vi "Teleop.vi"(10 "Match Info":T1={"Autonomous Elapsed Seconds"=0.0, "TeleOp Elapsed Seconds"=0.0, "Disabled Elapsed Seconds"=0.0, "Visited Autonomous"=FALSE, "Visited TeleOp"=FALSE, "Visited Disabled"=FALSE, "Autonomous Settings"={"Autonomous Style"=enum."Independent", "VI Refnum"=refnum}}, 11 "Call Context":T2) -> ()   [LabVIEW 2012]
doc: "This VI is called for each TeleOp packet received from the DS where the robot is not disabled. It is often used to read from the joysticks and update I/O or to update setpoints for timed control loops. It should complete and return within 20 milliseconds or it may miss DS packets."
uses:
  Robot Global Data.vi
  <vilib>/Rock Robotics/WPI/Solenoid/Deprecated/WPI_SolenoidSetBool.vi
  <vilib>/Rock Robotics/WPI/DriverStation/WPI_DriverStationMatch Info.ctl
  <vilib>/Rock Robotics/WPI/DriverStation/WPI_DriverStationDerivedRobotMode.ctl
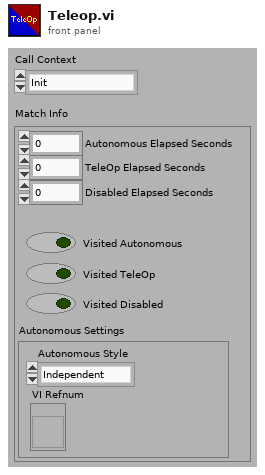
[diagram p1: front panel]
types:
  T1 = typedef "WPI_DriverStationMatch Info.ctl" = cluster{"Autonomous Elapsed Seconds":dbl, "TeleOp Elapsed Seconds":dbl, "Disabled Elapsed Seconds":dbl, "Visited Autonomous":bool, "Visited TeleOp":bool, "Visited Disabled":bool, "Autonomous Settings":cluster{"Autonomous Style":enum16{"Iterative", "Independent"}, "VI Refnum":refnum<vi>}}
  T2 = typedef "WPI_DriverStationDerivedRobotMode.ctl" = enum16{"Init", "Execute", "Stop"}
  T3 = typedef "WPI_DigitalInputDevRef.ctl" = cluster{"DevStatus":errorcluster, "DIO Channel":T4, "Digital Module":T5}
  T4 = typedef "FPGA_DIOChannel.ctl" = enum8{"DIO 1", "DIO 2", "DIO 3", "DIO 4", "DIO 5", "DIO 6", "DIO 7", "DIO 8", "DIO 9", "DIO 10", "DIO 11", "DIO 12", "DIO 13", "DIO 14", "Invalid"}
  T5 = typedef "FPGA_TypedefDigitalModule.ctl" = enum16{"Digital Module 1", "Digital Module 2"}
  T6 = typedef "WPI_MotorControlDeviceRef.ctl" = cluster{"DeviceStatus":errorcluster, "Type":enum16{"PWM", "CAN"}, "PWM":cluster{"Digital Module":T5, "PWM Channel":T7, "DeadBand":T8}, "CAN":cluster{"Device Number":u8, "Control Mode":T9, "Semaphore":T10, "Max Vout":dbl}, "Invert":bool, "TransformRef":T11, "InvTransformRef":T11}
  T7 = typedef "FPGA_DIOPWMChannel.ctl" = enum8{"PWM 1", "PWM 2", "PWM 3", "PWM 4", "PWM 5", "PWM 6", "PWM 7", "PWM 8", "PWM 9", "PWM 10", "Invalid"}
  T8 = typedef "WPI_PWMDeadband.ctl" = cluster{"Name":string, "maxPositivePwm":i32, "minPositivePwm":i32, "centerPwm":i32, "maxNegativePwm":i32, "minNegativePwm":i32, "angularRange":u16}
  T9 = typedef "WPI_CANJaguar_ControlMode.ctl" = enum8{"Percent VBus", "Current", "Speed", "Position", "Voltage"}
  T10 = typedef "Semaphore RefNum" = refnum<k1>
  T11 = typedef "WPI_PWMTransform_ConPane.ctl" = refnum<vi>
  T12 = typedef "WPI_JoystickDevRef.ctl" = cluster{"Device":T13}
  T13 = typedef "WPI_JoystickDeviceEnum.ctl" = enum16{"USB 1", "USB 2", "USB 3", "USB 4", "Kinect 1", "Kinect 2"}
  T14 = typedef "WPI_JoystickButtonState.ctl" = cluster{"Button 1":bool, "Button 2":bool, "Button 3":bool, "Button 4":bool, "Button 5":bool, "Button 6":bool, "Button 7":bool, "Button 8":bool, "Button 9":bool, "Button 10":bool, "Button 11":bool, "Button 12":bool}
  T15 = cluster{"axis 1 (x)":dbl, "axis 2 (y)":dbl, "axis 3 (throttle)":dbl, "axis 4":dbl, "axis 5":dbl, "axis 6":dbl}
  T16 = typedef "WPI_RobotDriveDevRef.ctl" = cluster{"DevStatus":errorcluster, "Motors[]":T6[], "Square Inputs":bool, "Max Output":dbl, "Isochronous":bool}
  T17 = typedef "WPI_SolenoidDevRef.ctl" = cluster{"DevStatus":errorcluster, "Solenoid Module":T18, "Forward Solenoid Channel":T19, "Reverse Solenoid Channel":T19}
  T18 = typedef "FPGA_TypedefSolenoidModule.ctl" = enum16{"Solenoid Module 1", "Solenoid Module 2"}
  T19 = typedef "WPI_SolenoidChannel.ctl" = enum8{"Solenoid 1", "Solenoid 2", "Solenoid 3", "Solenoid 4", "Solenoid 5", "Solenoid 6", "Solenoid 7", "Solenoid 8", "Invalid"}
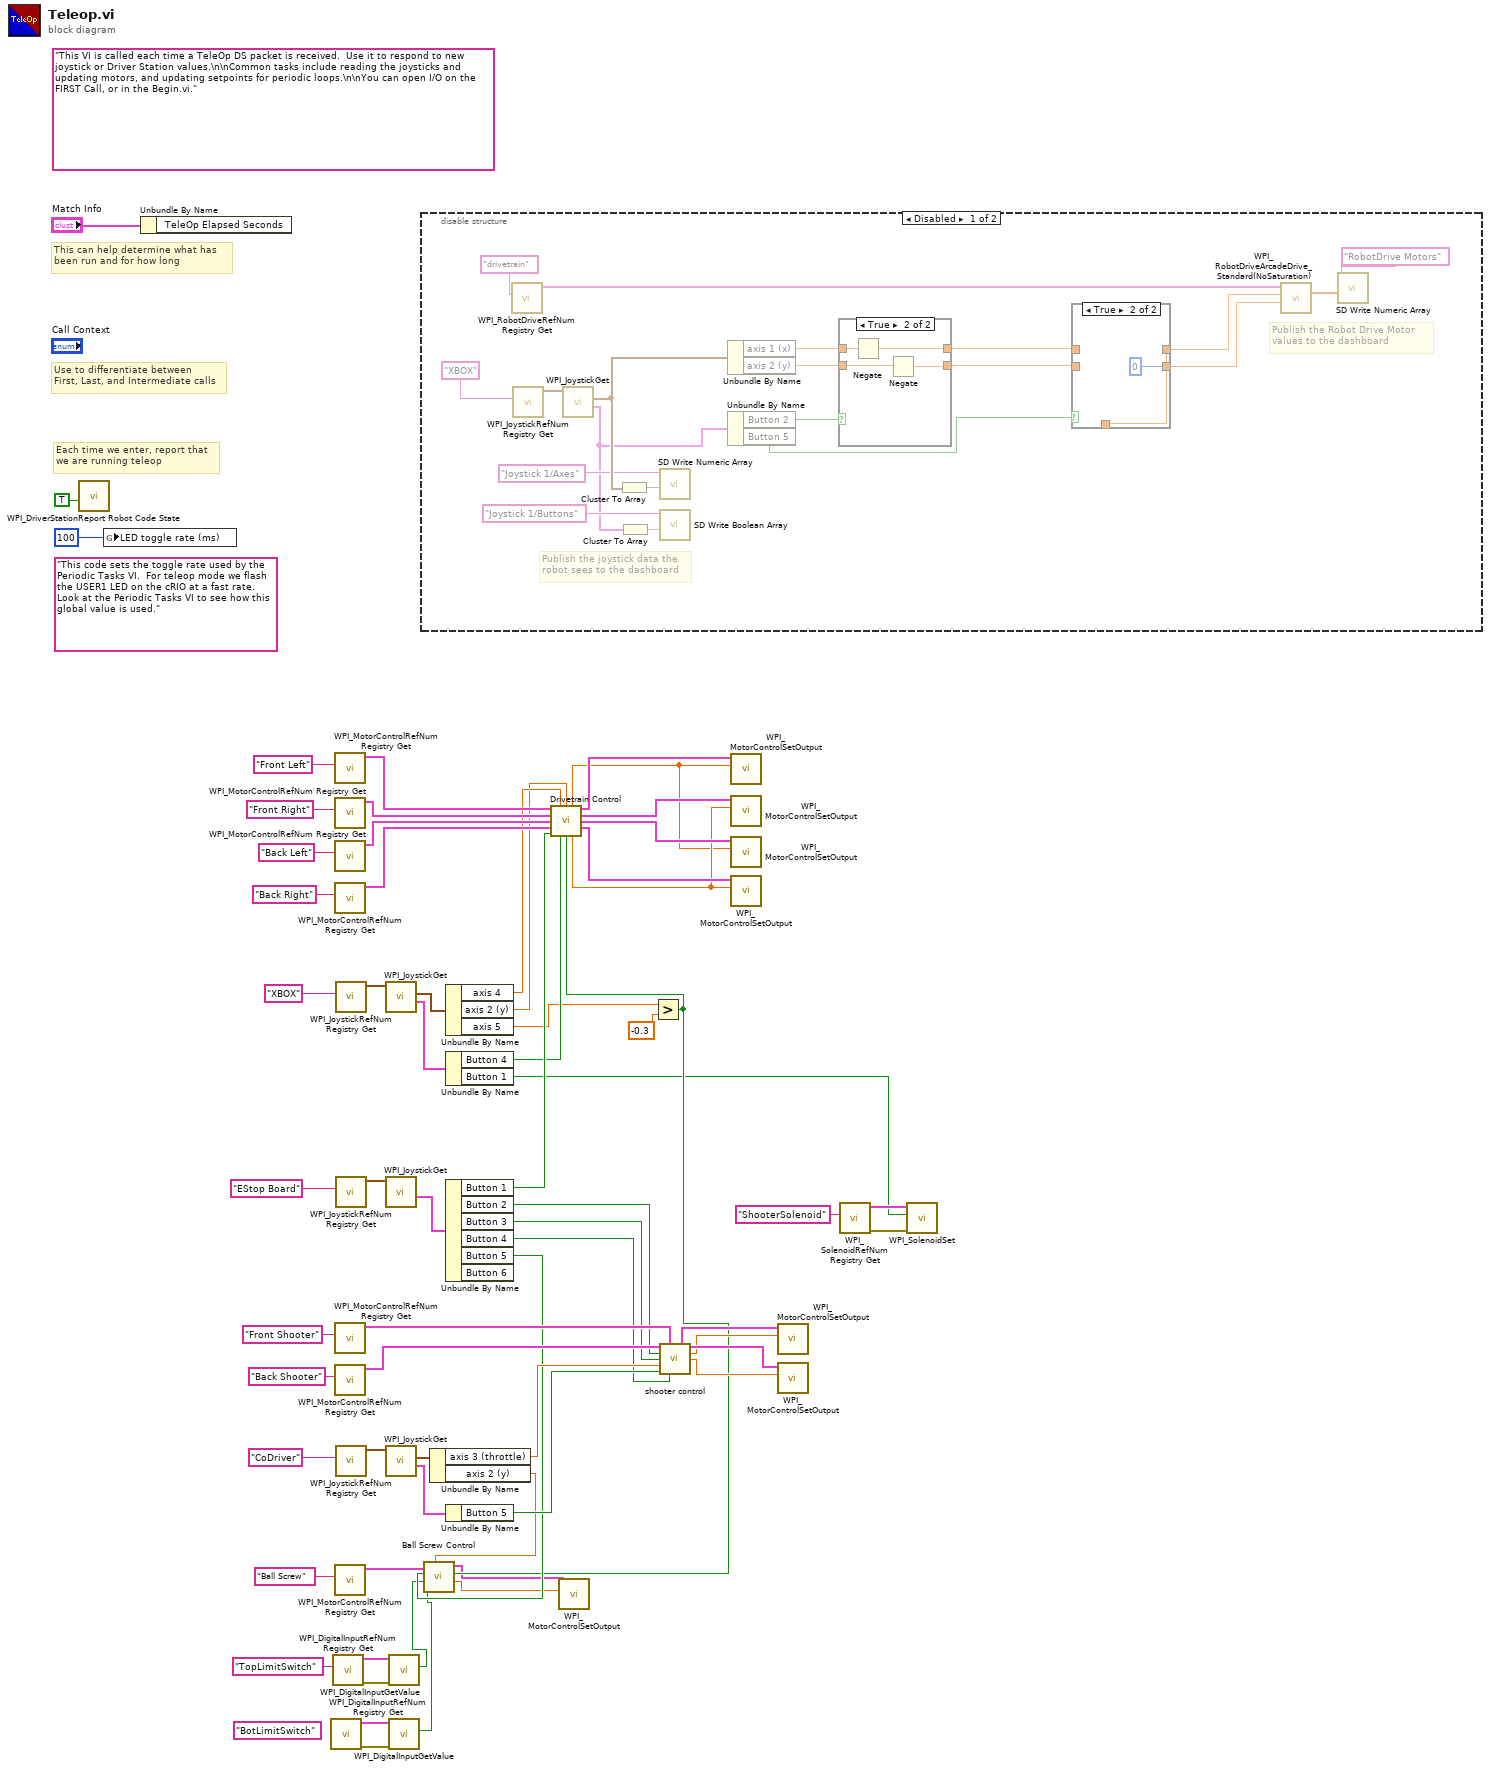
[diagram p0: block diagram]
diagram:
  (unwired) "BotLimitSwitch" ("refnum name")
  (unwired) "This code sets the toggle rate used by the Periodic Tasks VI.  For teleop mode we flash the USER1 LED on the cRIO at a fast rate.  Look at the Periodic Tasks VI to see how this global value is used."
  (unwired) "This VI is called each time a TeleOp DS packet is received.  Use it to respond to new joystick or Driver Station values.\n\nCommon tasks include reading the joysticks and updating motors, and updating setpoints for periodic loops.\n\nYou can open I/O on the FIRST Call, or in the Begin.vi."
  # "Each time we enter, report that\nwe are running teleop"
  # "Use to differentiate between\nFirst, Last, and Intermediate calls"
  # "This can help determine what has\nbeen run and for how long"
  n1 = call <vilib>:"WPI_DriverStationReport Robot Code State.vi"("TeleOp"=TRUE ("Autonomous")) -> ()  [unwired: 10 in, 1 out]
  n2 = global write "Robot Global Data.vi" "LED toggle rate (ms)"(u32 100 ("LED ms toggle rate")) -> ()
  n3 = Unbundle By Name("Match Info") -> ()  [unwired: 1 out]
  n4 = call <vilib>:"WPI_DigitalInputRefNum Registry Get.vi"() -> ("error out"=w14:errorcluster, "DigitalInputDevRef"=w13:T3)  [unwired: 10 in]
  n5 = call <vilib>:"WPI_DigitalInputRefNum Registry Get.vi"("refnum name"="TopLimitSwitch") -> ("error out"=w16:errorcluster, "DigitalInputDevRef"=w15:T3)  [unwired: 9 in]
  n6 = call <vilib>:"WPI_MotorControlRefNum Registry Get.vi"("refnum name"="Front Left") -> ("MotorControlDevRef"=w55:T6)  [unwired: 9 in, 1 out]
  n7 = call <vilib>:"WPI_MotorControlRefNum Registry Get.vi"("refnum name"="Front Right") -> ("MotorControlDevRef"=w54:T6)  [unwired: 9 in, 1 out]
  n8 = call <vilib>:"WPI_MotorControlRefNum Registry Get.vi"("refnum name"="Back Left") -> ("MotorControlDevRef"=w53:T6)  [unwired: 9 in, 1 out]
  n9 = call <vilib>:"WPI_MotorControlRefNum Registry Get.vi"("refnum name"="Back Right") -> ("MotorControlDevRef"=w52:T6)  [unwired: 9 in, 1 out]
  n10 = call <vilib>:"WPI_MotorControlRefNum Registry Get.vi"("refnum name"="Front Shooter") -> ("MotorControlDevRef"=w30:T6)  [unwired: 9 in, 1 out]
  n11 = call <vilib>:"WPI_MotorControlRefNum Registry Get.vi"("refnum name"="Back Shooter") -> ("MotorControlDevRef"=w31:T6)  [unwired: 9 in, 1 out]
  n12 = call <vilib>:"WPI_MotorControlRefNum Registry Get.vi"("refnum name"="Ball Screw") -> ("MotorControlDevRef"=w18:T6)  [unwired: 9 in, 1 out]
  n13 = call <vilib>:"WPI_JoystickRefNum Registry Get.vi"("refnum name"="XBOX") -> ("JoystickDevRef"=w50:T12)  [unwired: 1 in, 9 out]
  n14 = call <vilib>:"WPI_JoystickRefNum Registry Get.vi"("refnum name"="EStop Board") -> ("JoystickDevRef"=w40:T12)  [unwired: 1 in, 9 out]
  n15 = call <vilib>:"WPI_JoystickRefNum Registry Get.vi"("refnum name"="CoDriver") -> ("JoystickDevRef"=w44:T12)  [unwired: 1 in, 9 out]
  n16 = call <vilib>:"WPI_JoystickGet.vi"("JoystickDevRef"=w50) -> ("Buttons"=w46:T14, "Axes"=w49:T15)  [unwired: 1 in, 4 out]
  n17 = call <vilib>:"WPI_JoystickGet.vi"("JoystickDevRef"=w40) -> ("Buttons"=w39:T14)  [unwired: 1 in, 5 out]
  n18 = call <vilib>:"WPI_JoystickGet.vi"("JoystickDevRef"=w44) -> ("Buttons"=w42:T14, "Axes"=w43:T15)  [unwired: 1 in, 4 out]
  n19 = call <vilib>:"WPI_DigitalInputGetValue.vi"("error in (no error)"=w16, "DigitalInputDevRef"=w15) -> ("Value"=w12:bool)  [unwired: 7 in, 2 out]
  n20 = call <vilib>:"WPI_DigitalInputGetValue.vi"("error in (no error)"=w14, "DigitalInputDevRef"=w13) -> ("Value"=w11:bool)  [unwired: 7 in, 2 out]
  n21 = disable-structure shown="Disabled" {
    frame Disabled {
      # "Publish the Robot Drive Motor\nvalues to the dashboard"
      # "Publish the joystick data the\nrobot sees to the dashboard"
      n22 = call <vilib>:"WPI_RobotDriveRefNum Registry Get.vi"("refnum name"="drivetrain") -> ("RobotDriveDevRef"=w85:T16)  [unwired: 1 in, 9 out]
      n23 = call <vilib>:"WPI_JoystickRefNum Registry Get.vi"("refnum name"="XBOX") -> ("JoystickDevRef"=w83:T12)  [unwired: 1 in, 9 out]
      n24 = call <vilib>:"WPI_JoystickGet.vi"("JoystickDevRef"=w83) -> ("Buttons"=w75:T14, "Axes"=w80:T15)  [unwired: 1 in, 4 out]
      n25 = Cluster To Array(cluster=w80) -> (array=w79:dbl[])
      n26 = Cluster To Array(cluster=w75) -> (array=w82:bool[])
      n27 = call <vilib>:"SD Write Numeric Array.vi"("Numeric Array"=w79, "Name"="Joystick 1/Axes") -> ()  [unwired: 8 in, 2 out]
      n28 = call <vilib>:"SD Write Boolean Array.vi"("Boolean Array"=w82, "Name"="Joystick 1/Buttons") -> ()  [unwired: 8 in, 2 out]
      n29 = Unbundle By Name(w80) -> ("axis 1 (x)"=w73:dbl, "axis 2 (y)"=w72:dbl)
      n30 = Unbundle By Name(w75) -> ("Button 2"=w74:bool, "Button 5"=w71:bool)
      n31 = case shown="True" w74 {
        tunnel: [w92 w93] -> w69
        tunnel: w73 -> [w92 w96]
        tunnel: [w91 w94] -> w67
        tunnel: w72 -> [w91 w95]
        frame False {
        }
        frame True {
          n32 = Negate(x=w96) -> (-x=w93:dbl)
          n33 = Negate(x=w95) -> (-x=w94:dbl)
        }
      }
      n34 = case shown="True" w71 {
        tunnel: [w88 w89] -> w70
        tunnel: w69 -> [w88 _]
        tunnel: [w87 0] -> w68
        tunnel: w67 -> [w87 _]
        tunnel: [_ w89] -> w66
        frame False {
        }
        frame True {
        }
      }
      n35 = call <vilib>:"WPI_RobotDriveArcadeDrive_Standard(NoSaturation).vi"("Y axis value"=w68, "X axis value"=w70, "RobotDriveDevRef"=w85) -> ("Motor Values"=w76:dbl[])  [unwired: 1 in, 7 out]
      n36 = call <vilib>:"SD Write Numeric Array.vi"("Numeric Array"=w76, "Name"="RobotDrive Motors") -> ()  [unwired: 8 in, 2 out]
    }
    frame Enabled {
    }
  }
  n37 = Unbundle By Name(w43) -> ("axis 3 (throttle)"=w24:dbl, "axis 2 (y)"=w10:dbl)
  n38 = Unbundle By Name(w49) -> ("axis 4"=w48:dbl, "axis 2 (y)"=w47:dbl, "axis 5"=w8:dbl)
  n39 = Unbundle By Name(w46) -> ("Button 4"=w20:bool, "Button 1"=w1:bool)
  n40 = Unbundle By Name(w39) -> ("Button 1"=w32:bool, "Button 2"=w23:bool, "Button 3"=w22:bool, "Button 4"=w21:bool, "Button 5"=w17:bool)  [unwired: 1 out]
  n41 = Unbundle By Name(w42) -> ("Button 5"=w25:bool)
  n42 = Greater?(x=w8, y=-0.3) -> (0:w7:bool)
  n43 = call "Ball Screw Control.vi"("Target Button"=w7, "Joystick Axis"=w10, "Bot Limit"=w11, "Top Limit"=w12, "Closed Loop On/Off"=w17, "Ball Screw DevRef In"=w18) -> ("Motor Output"=w5:dbl, "Ball Screw DevRef Out"=w6:T6)  [unwired: 4 in]
  n44 = call "Drivetrain Control.vi"("Back Left DevRef In"=w55, "X Axis"=w48, "Y Axis"=w47, "Back Right DevRef In"=w54, "Front Left DevRef In"=w53, "Front Right DevRef In"=w52, "Closed Loop On/Off"=w32, "Drivetrain Reverse Button"=w20, "Trigger Axis"=w7) -> ("Left Motor Value"=w33:dbl, "Back Left DevRef Out"=w38:T6, "Back Right DevRef Out"=w37:T6, "Front Left DevRef Out"=w36:T6, "Front Right DevRef Out"=w35:T6, "Right Motor Value"=w34:dbl)  [unwired: 1 in]
  n45 = call <vilib>:"WPI_MotorControlSetOutput.vi"("Output"=w5, "MotorControlDevRef"=w6) -> ()  [unwired: 7 in, 3 out]
  n46 = call "shooter control.vi"("Back Shooter DevRef In"=w31, "Front Shooter DevRef In"=w30, "Closed Loop On/Off"=w23, "Power On/Off"=w22, "Joystick Throttle"=w24, "Target Button"=w25, "PyramidButton"=w21) -> ("Front Shooter DevRef Out"=w29:T6, "Back Shooter DevRef Out"=w28:T6, "FrontShooterOut"=w27:dbl, "BackShooterOut"=w26:dbl)  [unwired: 5 in]
  n47 = call <vilib>:"WPI_MotorControlSetOutput.vi"("Output"=w33, "MotorControlDevRef"=w38) -> ()  [unwired: 7 in, 3 out]
  n48 = call <vilib>:"WPI_MotorControlSetOutput.vi"("Output"=w34, "MotorControlDevRef"=w37) -> ()  [unwired: 7 in, 3 out]
  n49 = call <vilib>:"WPI_MotorControlSetOutput.vi"("Output"=w33, "MotorControlDevRef"=w36) -> ()  [unwired: 7 in, 3 out]
  n50 = call <vilib>:"WPI_MotorControlSetOutput.vi"("Output"=w34, "MotorControlDevRef"=w35) -> ()  [unwired: 7 in, 3 out]
  n51 = call <vilib>:"WPI_MotorControlSetOutput.vi"("Output"=w27, "MotorControlDevRef"=w29) -> ()  [unwired: 7 in, 3 out]
  n52 = call <vilib>:"WPI_MotorControlSetOutput.vi"("Output"=w26, "MotorControlDevRef"=w28) -> ()  [unwired: 7 in, 3 out]
  n53 = call <vilib>:"WPI_SolenoidRefNum Registry Get.vi"("refnum name"="ShooterSolenoid") -> ("error out"=w2:errorcluster, "SolenoidDevRef"=w3:T17)  [unwired: 9 in]
  n54 = call-poly <vilib>:"WPI_SolenoidSet.vi"("error in (no error)"=w2, "Value"=w1, "SolenoidDevRef"=w3) -> ()  [unwired: 7 in, 2 out]
